vi "CANOpen Addon Main Page.vi"(8 "error in (no error)":errorcluster, 11 "Node Ptr":T3 format="%.0x") -> (0 "error out":errorcluster)   [LabVIEW 2020, in "CANOpen Addon Custom Device.lvlib"]
uses:
  CANOpen Addon Custom Device.lvlib
  <vilib>/NI VeriStand/Custom Device API/Custom Device Item Ref.ctl
  Shared Code/CANOpen Interface Name.ctl
  <vilib>/CANopenLib/CANOPEN.llb/CANopen BaudRate.ctl
  <vilib>/NI VeriStand/Custom Device API/Custom Device File Dependency.ctl
  <vilib>/NI VeriStand/Custom Device API/Path Specification.ctl
  <vilib>/NI VeriStand/Custom Device API/Path Type.ctl
  <vilib>/NI VeriStand/Custom Device API/Custom Device Supported Target.ctl
  Shared Code/CANOpen Addon GUID Lookup Global.vi
  <vilib>/NI VeriStand/Custom Device API/Get Item Property (Variant).vi
  <vilib>/NI VeriStand/Custom Device API/Set Item Property (Variant).vi
  <vilib>/NI VeriStand/Custom Device API/Set Item Property (Path).vi
  <vilib>/NI VeriStand/Custom Device API/Custom Device API.lvlib
panel:
  in  "*Scan and print":bool caption="Scan connected devices on startup and print to screen."
  in  "*EDS File":path caption="EDS File"
  in  "*Enable SYNC":bool=TRUE caption="Synchronous"
  in  "*RIO Device":u16 caption="RIO Device"
  in  "Header 2":cluster{"Section Name":string}={"Section Name"="NI 9881 Support"}
  in  "*9881 Bitfile":path caption="Bitfile"
  in  "*Enable 9881":bool caption="Enable"
  in  "*Sync Period (ms)":i64=100 caption="Sync Period (ms) and CANopen device engine period"
  in  "SHDocVw.IWebBrowser2":refnum<k7>(container)
  in  "*Termination":bool=TRUE caption="Termination"
  in  "*Baud Rate":T1 caption="Baud Rate" items=["1 Mbit/s"=0, "800 kbit/s"=1, "500 kbit/s"=2, "250 kbit/s"=3, "125 kbit/s"=4, "50 kbit/s"=6, "20 kbit/s"=7, "10 kbit/s"=8]
  in  "*CANOpen Interface Name":T2 caption="CANOpen Interface Name" items=["CANopen01", "CANopen02", "CANopen03", "CANopen04", "CANopen05", "CANopen06", "CANopen07", "CANopen08", "CANopen09", "CANopen10", "CANopen11", "CANopen12", "CANopen13", "CANopen14", "CANopen15", "CANopen16", "CANopen17", "CANopen18", "CANopen19", "CANopen20", "CANopen21", "CANopen22", "CANopen23", "CANopen24", "CANopen25", "CANopen26", "CANopen27", "CANopen28", "CANopen29", "CANopen30", "CANopen31", "CANopen32"]
  in  "Header":cluster{"Section Name":string}={"Section Name"="CANOpen Addon Master Bus Settings"}
  in  "Name":string
  # "This can take up to 30 seconds"
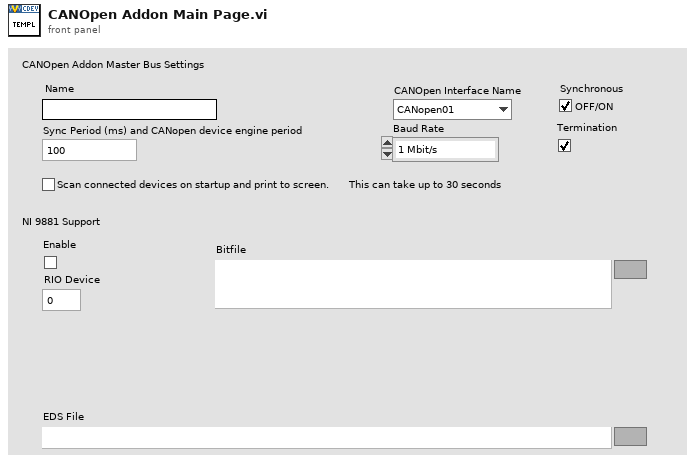
[diagram p1: front panel]
types:
  T1 = typedef "CANopen BaudRate.ctl" = u32
  T2 = typedef "CANOpen Addon Custom Device.lvlib/CANOpen Interface Name.ctl" = u32
  T3 = typedef "Custom Device API.lvlib/Custom Device Item Ref.ctl" = u64
  T4 = typedef "Custom Device API.lvlib/Custom Device Item Info.ctl" = cluster{"Name":string, "Is Channel":bool, "GUID":string, "Is Waveform":bool}
  T5 = typedef "Custom Device API.lvlib/Custom Device Supported Target.ctl" = enum16{"All", "PharLap", "VxWorks", "Windows", "Linux_32_ARM", "Linux_x64", "PharLap & Windows", "PharLap & VxWorks", "VxWorks & Windows"}
  T6 = typedef "Custom Device API.lvlib/Custom Device File Dependency.ctl" = cluster{"Source":T7, "RT Destination":path, "ForceDownload?":bool, "SupportedTarget":T5, "Version":string}
  T7 = typedef "Custom Device API.lvlib/Path Specification.ctl" = cluster{"Path":path, "Type":T8}
  T8 = typedef "Custom Device API.lvlib/Path Type.ctl" = enum16{"Absolute", "To Base", "To Common Data Dir", "To Application Data Dir"}
  T9 = typedef "Custom Device API.lvlib/Custom Device Commands.ctl" = enum16{"Default", "Item renamed", "Shutdown", "Dynamic button pressed"}
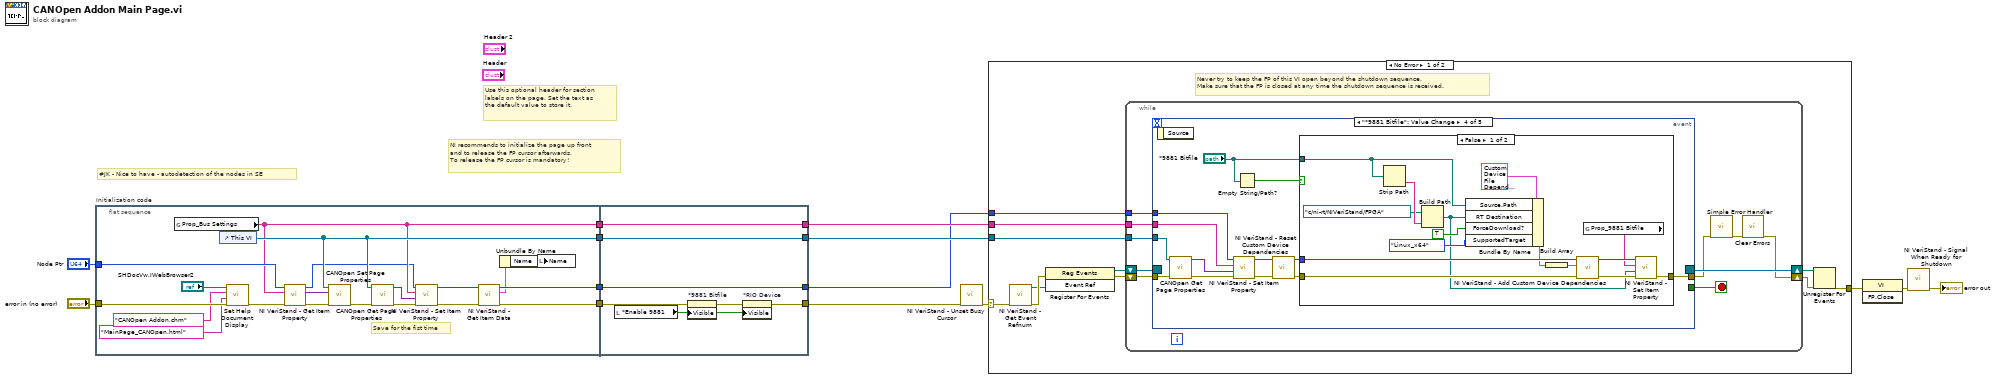
[diagram p0: block diagram]
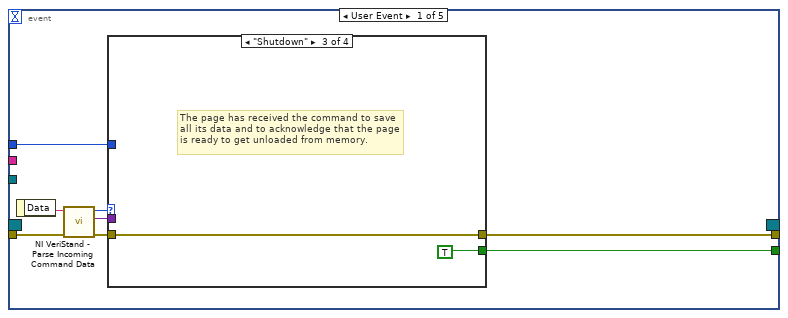
[diagram p2: hidden frame]
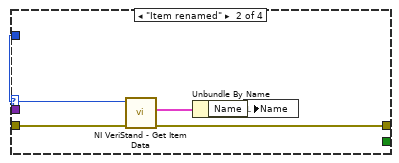
[diagram p4: hidden frame]
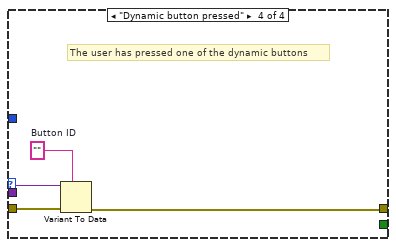
[diagram p5: hidden frame]
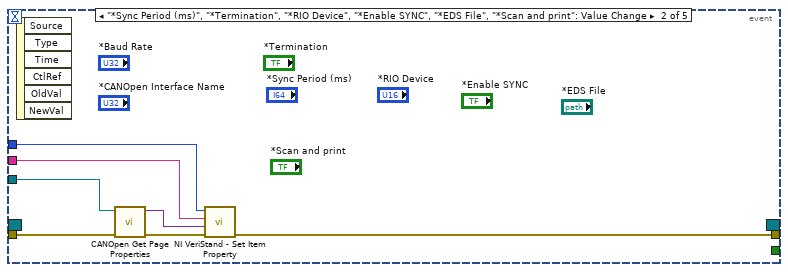
[diagram p6: hidden frame]
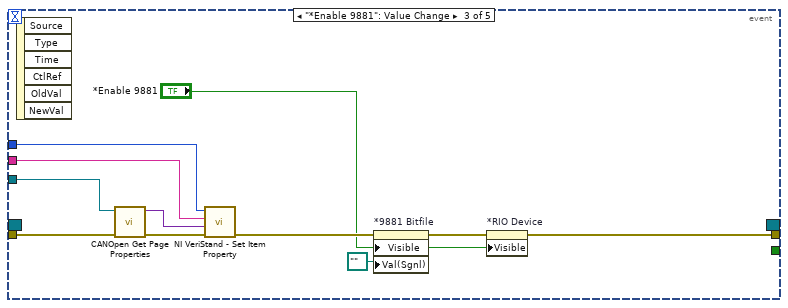
[diagram p7: hidden frame]
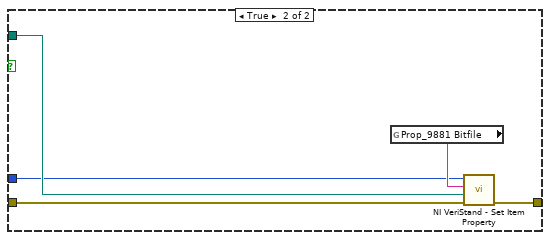
[diagram p8: hidden frame]
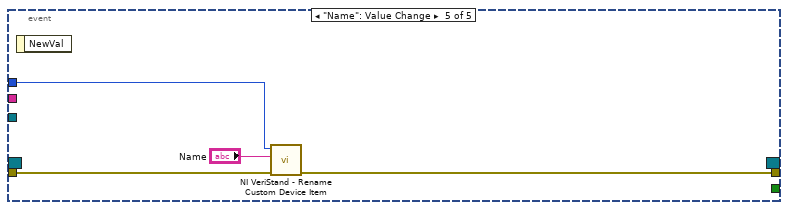
[diagram p9: hidden frame]
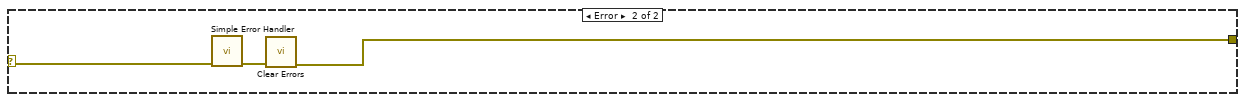
[diagram p10: hidden frame]
diagram:
  # "#JK - Nice to have - autodetection of the nodes in SE"
  # "Use this optional header for section labels on the page. Set the text as the default value to store it."
  # "NI recommends to initialize the page up front\nand to release the FP cursor afterwards.\nTo release the FP cursor is mandatory!"
  n1 = flat-sequence "Initialization code" {
    tunnel: "error in (no error)" -> [w30]
    tunnel: "Node Ptr" -> [w24]
    tunnel: [w31] -> w5
    tunnel: [w34] -> w4
    tunnel: [w17] -> w3
    tunnel: [w19] -> w2
    tunnel: [w40] -> w6
    tunnel: [w41] -> w7
    tunnel: [w35] -> w1
    tunnel: [w36] -> w10
    tunnel: w5 -> [w39]
    tunnel: w4 -> [w35]
    tunnel: w3 -> [w41]
    tunnel: w2 -> [w40]
    frame #0 {
      # "Save for the fist time"
      n2 = global read "CANOpen Addon GUID Lookup Global.vi" "Prop_Bus Settings"() -> (w17:string)
      n3 = control-ref of="This VI"() -> (w19:refnum<vi>)
      n4 = call "Set Help Document Display.vi"("error in (no error)"=w30, "HTML File"="MainPage_CANOpen.html", "Main CHM File"="CANOpen Addon.chm", "SHDocVw.IWebBrowser2"="SHDocVw.IWebBrowser2") -> ("error out"=w26:errorcluster)  [unwired: 7 in]
      n5 = call-poly <vilib>:"NI VeriStand - Get Item Property.vi"("error in (no error)"=w26, "Property Name"=w17, "Item Ref in"=w24) -> ("error out"=w25:errorcluster, "Value"=w23:variant, "Item Ref out"=w16:T3)  [unwired: 5 in, 1 out]
      n6 = call "CANOpen Set Page Properties.vi"("error in"=w25, "variant"=w23, "This VI"=w19) -> ("error out"=w20:errorcluster)  [unwired: 8 in]
      n7 = call "CANOpen Get Page Properties.vi"("error in (no error)"=w20, "This VI"=w19) -> ("error out"=w22:errorcluster, "Settings"=w21:variant)  [unwired: 8 in]
      n8 = call-poly <vilib>:"NI VeriStand - Set Item Property.vi"("error in (no error)"=w22, "Value"=w21, "Property Name"=w17, "Item Ref in"=w16) -> ("error out"=w18:errorcluster, "Item Ref out"=w15:T3)  [unwired: 5 in, 1 out]
      n9 = call <vilib>:"NI VeriStand - Get Item Data.vi"("error in (no error)"=w18, "Item Ref in"=w15) -> ("error out"=w31:errorcluster, "Item Info"=w33:T4, "Item Ref out"=w34:T3)  [unwired: 7 out]
      n10 = Unbundle By Name(w33) -> ("Name"=w32:string)
      n11 = local write "Name"(w32) -> ()
    }
    frame #1 {
      n12 = local read "*Enable 9881"() -> (w37:bool)
      n13 = property on="*9881 Bitfile" class="Path"(error in=w39, "Visible"=w37) -> (error out=w38:errorcluster)  [unwired: 1 in, 1 out]
      n14 = property on="*RIO Device" class="DigNum (strict)"(error in=w38, "Visible"=w37) -> (error out=w36:errorcluster)  [unwired: 1 in, 1 out]
    }
  }
  n15 = call <vilib>:"NI VeriStand - Unset Busy Cursor.vi"("error in (no error)"=w10) -> ("error out"=w9:errorcluster)  [unwired: 10 out]
  n16 = case shown="No Error" w9 {
    selector: w9 -> [w44 w140]
    tunnel: [w49 w138] -> w14
    tunnel: w1 -> [w45 _]
    tunnel: w7 -> [w43 _]
    tunnel: w6 -> [w42 _]
    frame No Error {
      # "Never try to keep the FP of this VI open beyond the shutdown sequence.\nMake sure that the FP is closed at any time the shutdown sequence is received."
      n17 = call <vilib>:"NI VeriStand - Get Event Refnum.vi"("error in (no error)"=w44) -> ("error out"=w52:errorcluster, "Event Ref"=w48:refnum<user-event>)  [unwired: 9 out]
      n18 = register-events(error in=w52, w48) -> (reference out=w46:refnum<event-registration>, error out=w47:errorcluster)  [unwired: 1 in]
      n19 = while {
        tunnel: w45 -> [w58]
        shift-right: [w55] -> w50
        shift-left: w47 -> [w61]
        shift-right: [w62] -> w51
        shift-left: w46 -> [w60]
        tunnel: w43 -> [w54]
        tunnel: w42 -> [w53]
        stop <- w59 stop-if-true
        n20 = event shown="[3] \"*9881 Bitfile\": Value Change" {
          selector: w60 -> [_ _ _ _ _]
          dyn-events: [_ _ _ _ _] -> w62
          timeout: _ -> [_ _ _ _ _]
          tunnel: w61 -> [w70 w89 w100 w106 w137]
          tunnel: [w66 _ _ _ _] -> w59
          tunnel: [w65 w85 w91 w111 w136] -> w57
          tunnel: w58 -> [w64 w86 w97 w104 w135]
          tunnel: w54 -> [_ w84 w96 w101 _]
          tunnel: w53 -> [_ w83 w95 w105 _]
          event User Event {
            n21 = event-data() -> ("Data"=w69:string)  [unwired: 1 out]
            n22 = call <vilib>:"NI VeriStand - Parse Incoming Command Data.vi"("error in (no error)"=w70, "Incoming data"=w69) -> ("error out"=w68:errorcluster, "Outgoing data"=w63:variant, "Action"=w67:T9)  [unwired: 7 out]
            n23 = case shown="\"Shutdown\"" w67 {
              tunnel: w68 -> [w71 w76 w77 w82]
              tunnel: [_ _ TRUE _] -> w66
              tunnel: [w71 w73 w77 w79] -> w65
              tunnel: w64 -> [_ w75 _ _]
              tunnel: w63 -> [_ _ _ w81]
              frame "Default", Default {
              }
              frame "Item renamed" {
                n24 = call <vilib>:"NI VeriStand - Get Item Data.vi"("error in (no error)"=w76, "Item Ref in"=w75) -> ("error out"=w73:errorcluster, "Item Info"=w74:T4)  [unwired: 8 out]
                n25 = Unbundle By Name(w74) -> ("Name"=w72:string)
                n26 = local write "Name"(w72) -> ()
              }
              frame "Shutdown" {
                # "The page has received the command to save all its data and to acknowledge that the page is ready to get unloaded from memory."
              }
              frame "Dynamic button pressed" {
                w80 = ""  # Button ID
                # "The user has pressed one of the dynamic buttons"
                n27 = Variant To Data(error in=w82, type=w80, Variant=w81) -> (error out=w79:errorcluster)  [unwired: 1 out]
              }
            }
          }
          event "*Sync Period (ms)", "*Termination", "*RIO Device", "*Enable SYNC", "*EDS File", "*Scan and print": Value Change {
            n28 = event-data() -> ()  [unwired: 7 out]
            n29 = call "CANOpen Get Page Properties.vi"("error in (no error)"=w89, "This VI"=w83) -> ("error out"=w88:errorcluster, "Settings"=w87:variant)  [unwired: 8 in]
            n30 = call-poly <vilib>:"NI VeriStand - Set Item Property.vi"("error in (no error)"=w88, "Value"=w87, "Property Name"=w84, "Item Ref in"=w86) -> ("error out"=w85:errorcluster)  [unwired: 5 in, 2 out]
          }
          event "*Enable 9881": Value Change {
            n31 = event-data() -> ()  [unwired: 7 out]
            n32 = call "CANOpen Get Page Properties.vi"("error in (no error)"=w100, "This VI"=w95) -> ("error out"=w99:errorcluster, "Settings"=w98:variant)  [unwired: 8 in]
            n33 = call-poly <vilib>:"NI VeriStand - Set Item Property.vi"("error in (no error)"=w99, "Value"=w98, "Property Name"=w96, "Item Ref in"=w97) -> ("error out"=w94:errorcluster)  [unwired: 5 in, 2 out]
            n34 = property on="*9881 Bitfile" class="Path"(error in=w94, "Visible"="*Enable 9881", "Val(Sgnl)"=path "" ("Value (Signaling)")) -> (error out=w92:errorcluster)  [unwired: 1 in, 1 out]
            n35 = property on="*RIO Device" class="DigNum (strict)"(error in=w92, "Visible"="*Enable 9881") -> (error out=w91:errorcluster)  [unwired: 1 in, 1 out]
          }
          event "*9881 Bitfile": Value Change {
            n36 = event-data() -> ()  [unwired: 2 out]
            n37 = call "CANOpen Get Page Properties.vi"("error in (no error)"=w106, "This VI"=w105) -> ("error out"=w108:errorcluster, "Settings"=w107:variant)  [unwired: 8 in]
            n38 = call-poly <vilib>:"NI VeriStand - Set Item Property.vi"("error in (no error)"=w108, "Value"=w107, "Property Name"=w101, "Item Ref in"=w104) -> ("error out"=w103:errorcluster, "Item Ref out"=w102:T3)  [unwired: 5 in, 1 out]
            n39 = Empty String/Path?(string/path="*9881 Bitfile") -> (empty?=w109:bool)
            n40 = call <vilib>:"NI VeriStand - Reset Custom Device Dependencies.vi"("error in (no error)"=w103, "Device Ref in"=w102) -> ("error out"=w113:errorcluster, "Device Ref out"=w112:T3)  [unwired: 8 in]
            n41 = case shown="False" w109 {
              tunnel: w113 -> [w128 w132]
              tunnel: w112 -> [w127 w129]
              tunnel: [w117 w131] -> w111
              tunnel: "*9881 Bitfile" -> [w119 w130]
              frame False {
                n42 = Strip Path(path=w119) -> (name=w121:string)  [unwired: 1 out]
                n43 = Build Path(base path=path "c:/ni-rt/NIVeriStand/FPGA" ("RT Destination"), name or relative path=w121) -> (appended path=w115:path)
                n44 = Bundle By Name(cluster=T6 {"Source"={"Path"=path "", "Type"=enum."Absolute"}, "RT Destination"=path "", "ForceDownload?"=FALSE, "SupportedTarget"=enum."PharLap", "Version"=""} ("Dependency"), "Source.Path"=w119, "RT Destination"=w115, "ForceDownload?"=TRUE, "SupportedTarget"=Custom_Device_Supported_Target."Linux_x64") -> (w125:T6)
                n45 = Build Array(w125) -> (w124:T6[])
                n46 = call <vilib>:"NI VeriStand - Add Custom Device Dependencies.vi"("error in (no error)"=w128, "Dependencies"=w124, "Device Ref in"=w127) -> ("error out"=w118:errorcluster, "Device Ref out"=w116:T3)  [unwired: 7 in]
                n47 = global read "CANOpen Addon GUID Lookup Global.vi" "Prop_9881 Bitfile"() -> (w114:string)
                n48 = call-poly <vilib>:"NI VeriStand - Set Item Property.vi"("error in (no error)"=w118, "Value"=w115, "Property Name"=w114, "Item Ref in"=w116) -> ("error out"=w117:errorcluster)  [unwired: 5 in, 2 out]
              }
              frame True {
                n49 = global read "CANOpen Addon GUID Lookup Global.vi" "Prop_9881 Bitfile"() -> (w133:string)
                n50 = call-poly <vilib>:"NI VeriStand - Set Item Property.vi"("error in (no error)"=w132, "Value"=w130, "Property Name"=w133, "Item Ref in"=w129) -> ("error out"=w131:errorcluster)  [unwired: 5 in, 2 out]
              }
            }
          }
          event "Name": Value Change {
            n51 = event-data() -> ()  [unwired: 2 out]
            n52 = call <vilib>:"NI VeriStand - Rename Custom Device Item.vi"("error in (no error)"=w137, "New Name"="Name", "Item Ref in"=w135) -> ("error out"=w136:errorcluster)  [unwired: 1 in, 7 out]
          }
        }
        n53 = call <vilib>:"Simple Error Handler.vi"("error in (no error)"=w57) -> ("error out"=w56:errorcluster)  [unwired: 1 in, 7 out]
        n54 = call <vilib>:"Clear Errors.vi"("error in (no error)"=w56) -> ("error out"=w55:errorcluster)  [unwired: 1 in, 5 out]
      }
      n55 = Unregister For Events(event registration refnum=w51, error in=w50) -> (error out=w49:errorcluster)
    }
    frame Error {
      n56 = call <vilib>:"Simple Error Handler.vi"("error in (no error)"=w140) -> ("error out"=w139:errorcluster)  [unwired: 1 in, 7 out]
      n57 = call <vilib>:"Clear Errors.vi"("error in (no error)"=w139) -> ("error out"=w138:errorcluster)  [unwired: 1 in, 5 out]
    }
  }
  n58 = invoke class="VI" method="FP.Close"(error in=w14) -> (error out=w13:errorcluster)  [unwired: 2 in, 2 out]
  n59 = call <vilib>:"NI VeriStand - Signal When Ready for Shutdown.vi"("error in (no error)"=w13) -> ("error out"=→"error out":errorcluster)  [unwired: 10 out]
